vi "PCAN_GetLaserPower.vi"(2 "Position":dbl, 3 "Laser No":i16, 4 "CAN Adress":u32, 5 "Extra Wait":bool=TRUE) -> (0 "Error ?":bool, 1 "Intensity (a.u.)":dbl)   [LabVIEW 2013]
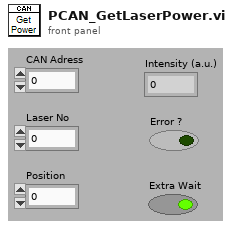
[diagram p1: front panel]
types:
  T1 = enum8{"STD, NO RTR", "STD,RTR", "XTD, NO RTR", "XTD, RTR"}
  T2 = cluster{"CAN Adress":u32, "MSG type":enum8{"STD, NO RTR", "STD,RTR", "XTD, NO RTR", "XTD, RTR"}, "LEN 3":u8, "Array":u8[]}
  T3 = cluster{"ID":u32, "MSG type":enum8{"STD, NO RTR", "STD,RTR", "XTD, NO RTR", "XTD, RTR"}, "LEN":u8, "DATA":u8[]}
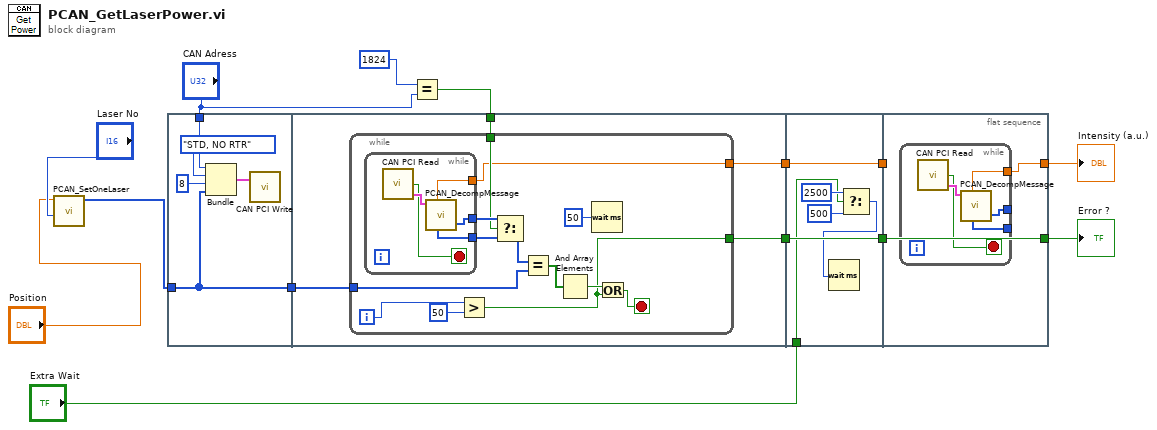
[diagram p0: block diagram]
diagram:
  n1 = call "PCAN_SetOneLaser.vi"("Laser No"="Laser No", "Value"="Position") -> ("Array"=w8:u8[])  [unwired: 8 in]
  n2 = flat-sequence {
    tunnel: "CAN Adress" -> [w18]
    tunnel: w8 -> [w15]
    tunnel: [w15] -> w14
    tunnel: w2 -> [w21]
    tunnel: w14 -> [w22]
    tunnel: [w23] -> w13
    tunnel: [w20] -> w12
    tunnel: w13 -> [w47]
    tunnel: [w47] -> w11
    tunnel: w12 -> [w46]
    tunnel: [w46] -> w10
    tunnel: "Extra Wait" -> [w42]
    tunnel: [w48] -> w6
    tunnel: [w49] -> w5
    tunnel: w11 -> [w49]
    tunnel: w10 -> [_]
    frame #0 {
      n3 = Bundle("CAN Adress"=w18, "MSG type"=T1."STD, NO RTR", "LEN 3"=u8 8, "Array"=w15) -> (w19:T2)  [unwired: 1 in]
      n4 = call "CAN PCI Write.vi"("CAN_Message"=w19) -> ()  [unwired: 2 in, 1 out]
    }
    frame #1 {
      n5 = while {
        tunnel: w22 -> [w31]
        tunnel: w21 -> [w33]
        tunnel: [w25] -> w23
        tunnel: [w24] -> w20
        i -> [w29]
        stop <- w26 stop-if-true
        n6 = while {
          tunnel: [w40] -> w24
          tunnel: [w38] -> w35
          tunnel: [w37] -> w34
          stop <- w39 stop-if-true
          n7 = call "CAN PCI Read.vi"() -> ("RcvQueueEmpty"=w39:bool, "CAN_Message out"=w41:T3)  [unwired: 1 in, 1 out]
          n8 = call "PCAN_DecompMessage.vi"("CAN_Message out"=w41) -> ("Laser 1-4"=w38:u8[], "Laser 5-8"=w37:u8[], "Intensity (a.u.)"=w40:dbl)  [unwired: 3 in, 5 out]
        }
        n9 = Greater?(x=w29, y=50) -> (0:w25:bool)
        n10 = Select(t=w35, s=w33, f=w34) -> (s? t:f=w32:u8[])
        n11 = Equal?(x=w32, y=w31) -> (x = y?=w30:bool[])
        n12 = And Array Elements(Boolean array=w30) -> (logical AND=w27:bool)
        n13 = Wait (ms)(milliseconds to wait=u32 50) -> ()  [unwired: 1 out]
        n14 = Or(x=w27, y=w25) -> (x .or. y?=w26:bool)
      }
    }
    frame #2 {
      n15 = Select(t=u32 2500 ("milliseconds to wait"), s=w42, f=u32 500 ("milliseconds to wait")) -> (s? t:f=w43:u32)
      n16 = Wait (ms)(milliseconds to wait=w43) -> ()  [unwired: 1 out]
    }
    frame #3 {
      n17 = while {
        tunnel: [w53] -> w48
        tunnel: [w51] -> _
        tunnel: [w50] -> _
        stop <- w52 stop-if-true
        n18 = call "CAN PCI Read.vi"() -> ("RcvQueueEmpty"=w52:bool, "CAN_Message out"=w54:T3)  [unwired: 1 in, 1 out]
        n19 = call "PCAN_DecompMessage.vi"("CAN_Message out"=w54) -> ("Laser 1-4"=w51:u8[], "Laser 5-8"=w50:u8[], "Intensity (a.u.)"=w53:dbl)  [unwired: 3 in, 5 out]
      }
    }
  }
  n20 = Equal?(x=u32 1824, y="CAN Adress") -> (x = y?=w2:bool)
  "Intensity (a.u.)" <- w6
  "Error ?" <- w5
